vi "Convert To Subpanel Tag.vi"(8 "error in":errorcluster, 10 "subpanel UID":i32, 11 "owning VI name":string) -> (0 "error out":errorcluster, 3 "subpanel tag":string)   [LabVIEW 2010, in "NI_SE_Config Front Panel Layout.lvlib"]
uses:
  NI_SE_Config Front Panel Layout.lvlib
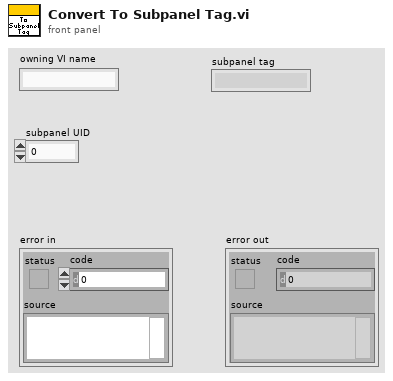
[diagram p1: front panel]
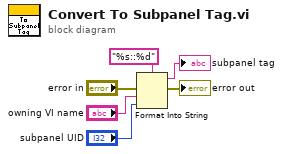
[diagram p0: block diagram]
diagram:
  n1 = Format Into String(format string="%s::%d", error in="error in", "owning VI name", "subpanel UID") -> (resulting string=→"subpanel tag":string, error out=→"error out":errorcluster)  [unwired: 1 in]
